vi "Midterm.vi"() -> ()   [LabVIEW 2023]
uses:
  <vilib>/express/express analysis/Spectral/Block/exnSpectralBlock spectral measurements RMS poly.vi
  <vilib>/express/express analysis/Spectral/Block/exnSpectralBlock spectral measurements RMS DDT.vi
  <vilib>/express/express analysis/Spectral/XNode/ExpressSpectralMeasurementsBlockNode.xnode
  <vilib>/Analysis/NI_AALPro.lvlib
panel:
  out "FFT RMS":dynamicdata(graph)
  out "Corresponding Frequency (Hz)":dbl
  out "FFT Max Amplitude":dbl
  out "?":dbl
  out "Original Sound Data":dynamicdata(graph)
  in  "Duration (s)":dbl=1.0
  # "Spectrum Analyzer"
  # "Duration of the Recording"
  # "Total Sound Pressure (in dB)"
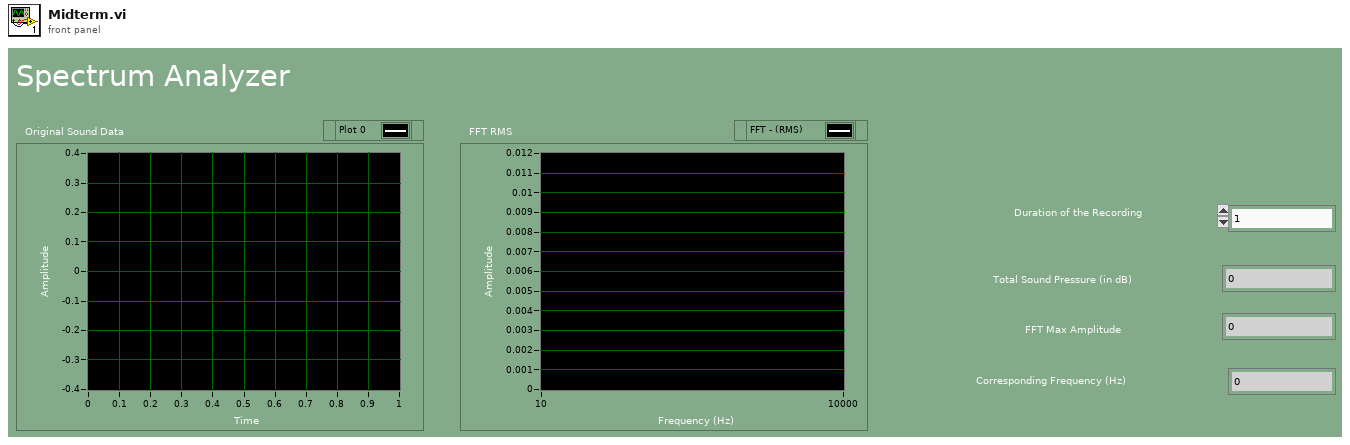
[diagram p1: front panel]
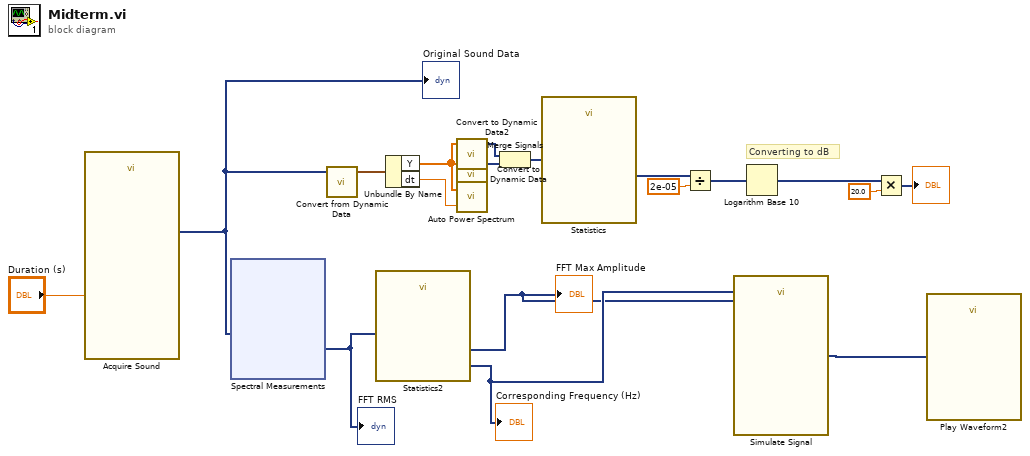
[diagram p0: block diagram]
diagram:
  # "Converting to dB"
  n1 = call "Acquire Sound"("Duration (s)"="Duration (s)") -> ("Data"=w5:dynamicdata)  [unwired: 17 in, 1 out]
  "Original Sound Data" <- w5
  n2 = xnode "Spectral Measurements"("Signals"=w5) -> ("FFT - (RMS)"=w4:dynamicdata)  [unwired: 1 in, 2 out]
  "FFT RMS" <- w4
  n3 = call "Convert from Dynamic Data"("Dynamic Data Type"=w5) -> ("Waveform"=w17:waveform(dbl))  [unwired: 3 in]
  n4 = call "Statistics2"("Signals"=w4) -> ("Time of Maximum"=w3:dynamicdata, "Maximum"=w2:dynamicdata)  [unwired: 24 in, 1 out]
  "FFT Max Amplitude" <- w2
  "Corresponding Frequency (Hz)" <- w3
  n5 = Unbundle By Name(w17) -> ("Y"=w12:dbl[], "dt"=w18:dbl)
  n6 = call "Convert to Dynamic Data2"("Array"=w12) -> ("Dynamic Data Type"=w15:dynamicdata)  [unwired: 3 in]
  n7 = call "Convert to Dynamic Data"("Array"=w12) -> ("Dynamic Data Type"=w11:dynamicdata)  [unwired: 3 in]
  n8 = call <vilib>:"Auto Power Spectrum.vi"("dt"=w18, "Signal (V)"=w12) -> ()  [unwired: 2 out]
  n9 = Merge Signals(w15, w11) -> (w13:dynamicdata)
  n10 = call "Statistics"("Signals"=w13) -> ("RMS"=w10:dynamicdata)  [unwired: 25 in, 1 out]
  n11 = Divide(x=w10, y=2e-05) -> (x/y=w9:dynamicdata)
  n12 = call "Simulate Signal"("Frequency"=w3, "Amplitude"=w2) -> ("Sine"=w1:dynamicdata)  [unwired: 12 in, 1 out]
  n13 = Logarithm Base 10(1:w9) -> (0:w16:dynamicdata)
  n14 = Multiply(x=w16, y=20.0) -> (x*y=→"?":dynamicdata)
  n15 = call "Play Waveform2"("Data"=w1) -> ()  [unwired: 18 in, 1 out]
